vi "Going for Container set.vi"   [LabVIEW 2014]
uses:
  TypeDefs/SRE Enum.ctl
  <vilib>/Rock Robotics/Network Tables/SD Read Number.vi
  Support Code/Robot Global Data.vi
types:
  T1 = enum16{"High", "Middle", "Low", "Really Low", "Stopped"}
  T2 = typedef "SRE Enum.ctl" = enum16{"Start", "Run", "End"}
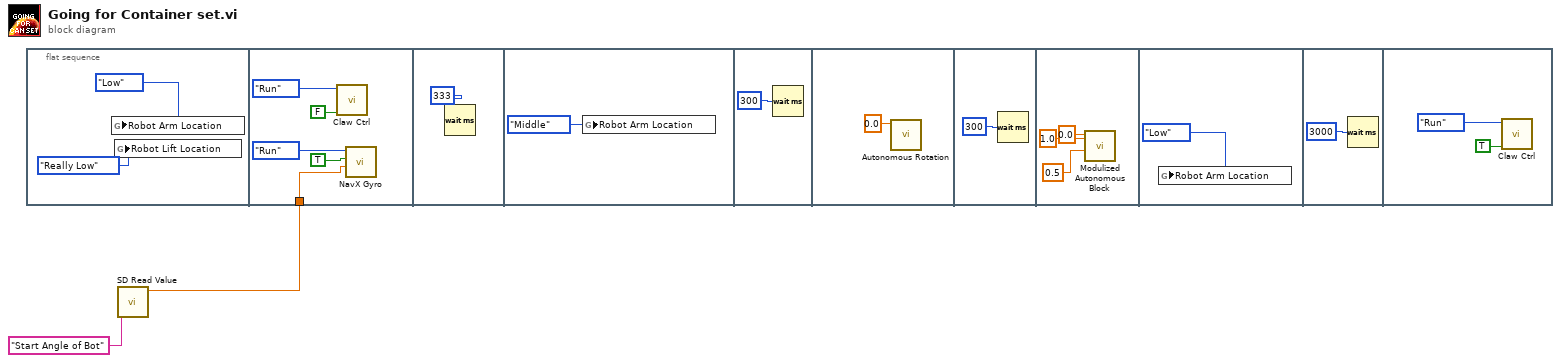
[diagram p0: block diagram]
diagram:
  n1 = flat-sequence {
    tunnel: w1 -> [w5]
    frame #0 {
      n2 = global write "Robot Global Data.vi" "Robot Arm Location"(enum16{"High", "Middle", "Low", "Noodle"}."Low" ("Robot Arm Location")) -> ()
      n3 = global write "Robot Global Data.vi" "Robot Lift Location"(T1."Really Low" ("Robot Lift Location")) -> ()
    }
    frame #1 {
      n4 = call "Claw Ctrl.vi"("Open/Close"=FALSE, "Enum"=SRE_Enum."Run") -> ()  [unwired: 10 in]
      n5 = call "NavX Gyro.vi"("Set To"=w5, "Reset"=TRUE, "Enum"=SRE_Enum."Run") -> ()  [unwired: 7 in, 2 out]
    }
    frame #2 {
      n6 = Wait (ms)(milliseconds to wait=u32 333) -> ()  [unwired: 1 out]
    }
    frame #3 {
      n7 = global write "Robot Global Data.vi" "Robot Arm Location"(enum16{"High", "Middle", "Low", "Noodle"}."Middle" ("Robot Arm Location")) -> ()
    }
    frame #4 {
      n8 = Wait (ms)(milliseconds to wait=u32 300) -> ()  [unwired: 1 out]
    }
    frame #5 {
      n9 = call "Autonomous Rotation.vi"("Angle"=0.0) -> ()  [unwired: 11 in]
    }
    frame #6 {
      n10 = Wait (ms)(milliseconds to wait=u32 300) -> ()  [unwired: 1 out]
    }
    frame #7 {
      n11 = call "Modulized Autonomous Block.vi"("Power"=0.5, "run time in seconds"=1.0, "Direction"=0.0) -> ()  [unwired: 8 in, 1 out]
    }
    frame #8 {
      n12 = global write "Robot Global Data.vi" "Robot Arm Location"(enum16{"High", "Middle", "Low", "Noodle"}."Low" ("Robot Arm Location")) -> ()
    }
    frame #9 {
      n13 = Wait (ms)(milliseconds to wait=u32 3000) -> ()  [unwired: 1 out]
    }
    frame #10 {
      n14 = call "Claw Ctrl.vi"("Open/Close"=TRUE, "Enum"=SRE_Enum."Run") -> ()  [unwired: 10 in]
    }
  }
  n15 = call-poly <vilib>:"SD Read Value.vi"("Name"="Start Angle of Bot") -> ("Numeric"=w1:dbl)  [unwired: 8 in, 2 out]
